vi "Rcycle(SubVI).vi"(1 "N cycles":dbl, 2 "Cycling\ntemperature\nto K factors":u16) -> (0 "Rcycle":dbl)   [LabVIEW 2017]
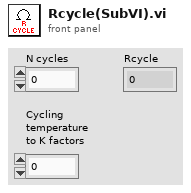
[diagram p1: front panel]
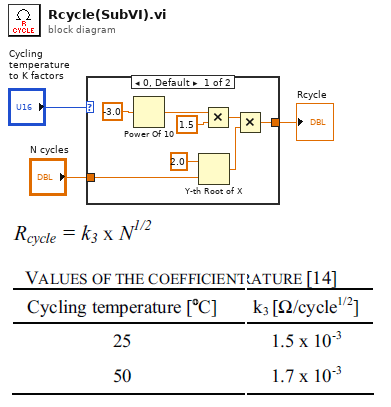
[diagram p0: block diagram]
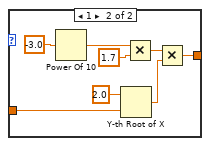
[diagram p2: hidden frame]
diagram:
  n1 = case shown="0, Default" "Cycling\ntemperature\nto K factors" {
    tunnel: "N cycles" -> [w10 w13]
    tunnel: [w4 w12] -> w3
    frame 0, Default {
      n2 = Power Of 10(x=-3.0) -> (10^x=w7:dbl)
      n3 = Y-th Root of X(1:w10, 2:2.0 ("y")) -> (0:w9:dbl)
      n4 = Multiply(x=w7, y=1.5) -> (x*y=w5:dbl)
      n5 = Multiply(x=w5, y=w9) -> (x*y=w4:dbl)
    }
    frame 1 {
      n6 = Power Of 10(x=-3.0) -> (10^x=w16:dbl)
      n7 = Y-th Root of X(1:w13, 2:2.0 ("y")) -> (0:w18:dbl)
      n8 = Multiply(x=w16, y=1.7) -> (x*y=w14:dbl)
      n9 = Multiply(x=w14, y=w18) -> (x*y=w12:dbl)
    }
  }
  "Rcycle" <- w3
